vi "ArbitraryPlane_miniscan_Generator.vi"(8 "error in":errorcluster, 9 "Main Zoom":dbl, 10 "Frame Size":i32=200, 11 "Input data":T1(array[cluster])=[{"X start"=25.0, "Y start"=55.0, "Z start"=8.0}, {"X start"=96.0, "Y start"=109.0, "Z start"=5.0}, {"X start"=185.0, "Y start"=99.0, "Z start"=-10.0}]) -> (0 "error out":errorcluster, 1 "XYZ Stop Norm":cluster{"X":sgl, "Y":sgl, "Z":sgl}[](array[cluster]), 2 "XYZ Start Norm":cluster{"X":sgl, "Y":sgl, "Z":sgl}[](array[cluster]), 3 "Corners of Plane":dbl[][](array[numeric]), 4 "Number of pixels in single X miniscan":i32)   [LabVIEW 2020]
uses:
  Global Variables/gl_UI Ctrl Refs.vi
panel:
  out "XYZ Stop":cluster{"X":sgl, "Y":sgl, "Z":sgl}[](array[cluster])
  out "XYZ Start":cluster{"X":sgl, "Y":sgl, "Z":sgl}[](array[cluster])
  out "pixels in  tilted miniscan":sgl[](array[numeric])
  out "Debugging indicator":cluster{sgl, sgl}[](array[cluster])
  out "Number of miniscans":i32
  out "Ystop-Ystart":i32[](array[numeric])
  out "stops":sgl[][](array[numeric])
  out "starts":sgl[][](array[numeric])
  out "Number of pixels in each X miniscan":i32[](array[numeric])
  out "Path":path
  out "P3 (xyz)":dbl[](array[numeric])
  out "P2 (xyz)":dbl[](array[numeric])
  out "P1 (xyz)":dbl[](array[numeric])
  # "Columns are POI\n4 POI one for each rectangle corner."
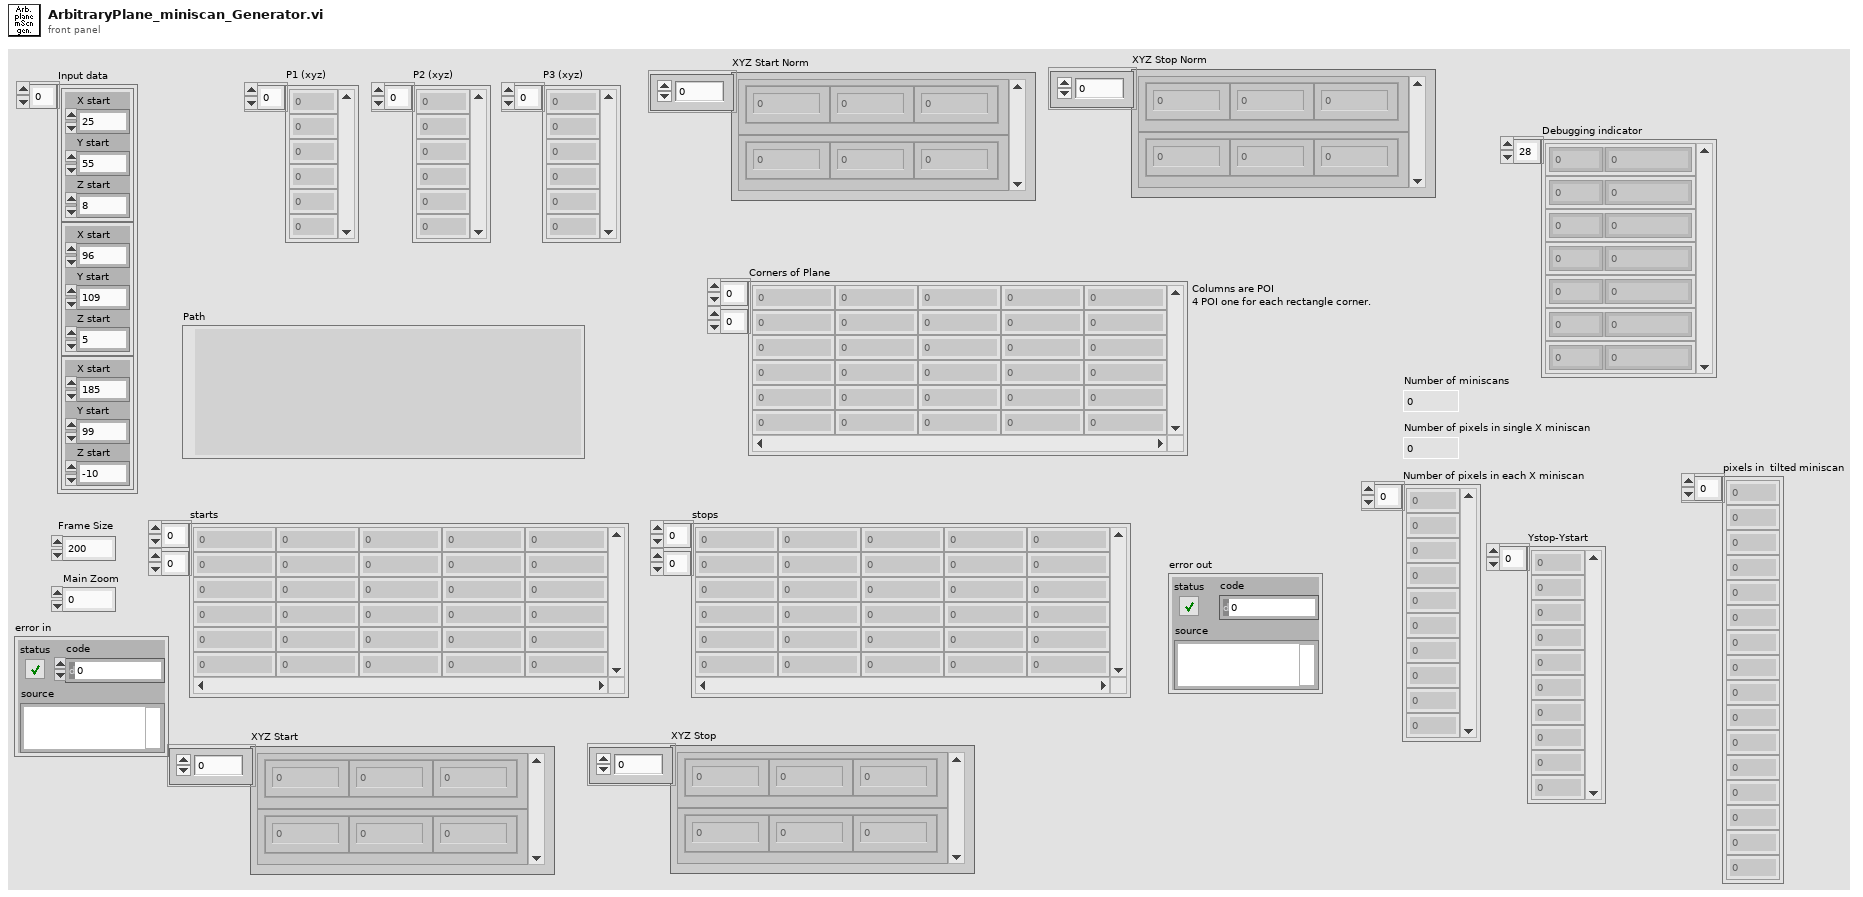
[diagram p1: front panel]
types:
  T1 = cluster{"X start":dbl, "Y start":dbl, "Z start":dbl}[]
  T2 = cluster{"X start":dbl, "Y start":dbl, "Z start":dbl}
  T3 = typedef "UI ctrl refs cluster.ctl" = cluster{"Top level VI path":path, "Top level VI ref":refnum<vi>, "User menu ref":refnum<k9>, "Sub Panel control":refnum<vi>, "Imaging Param Tab":refnum<vi>, "Occurrence-Start drivers":refnum<k4>, "Occurrence-Speed logging initialised":refnum<k4>, "Occurrence-XYZ stage initialised":refnum<k4>, "Exit button":refnum<vi>, "Status ind":refnum<vi>, "Set as origin":refnum<vi>, "Speed Logging":refnum<vi>, "Time Lapse":refnum<vi>, "Live Imaging":refnum<vi>, "AOL Z Stack":refnum<vi>, "Motor Z Stack":refnum<vi>, "Funct Acq button":refnum<vi>, "Hard Shutter":refnum<vi>, "Virtual Shutter":refnum<vi>, "Laser Power":refnum<vi>, "AOL Mode":refnum<vi>, "Frame Size":refnum<vi>, "Field of View":refnum<vi>, "Dwell Time":refnum<vi>, "Zoom":refnum<vi>, "AOL Z":refnum<vi>, "Objective":refnum<vi>, "Axis":refnum<vi>, "Paths & Names":refnum<vi>, "Experiment folder path (ind.)":refnum<vi>, "Last State (Ind.)":refnum<vi>, "Averages":refnum<vi>, "Angle (degrees)":refnum<vi>, "X centre":refnum<vi>, "Y centre":refnum<vi>, "Plane Mode":refnum<vi>, "# Planes":refnum<vi>, "Z Start":refnum<vi>, "Z Stop":refnum<vi>, "Z Step":refnum<vi>, "PMT 1":refnum<vi>, "PMT 2":refnum<vi>, "Stage XYZ Position":refnum<vi>, "Pockels@Z Start":refnum<vi>, "Pockels@Z Stop":refnum<vi>, "Obtain Z Start":refnum<vi>, "Obtain Z Stop":refnum<vi>, "Live stim.trig.period":refnum<vi>, "Live stim.trig.enable":refnum<vi>, "Movement Correction":refnum<vi>, "Load Reference Image":refnum<vi>, "XY Stage Move":refnum<vi>, "MovCor Cluster":refnum<vi>, "RefDAQParam":refnum<vi>, "Funct. Acq. Pockels Modulation":refnum<vi>, "Ref Laser Power":refnum<vi>, "Enable Video Recording":refnum<vi>, "Video Record-Live Imaging":refnum<vi>, "Video Record-Funct acq":refnum<vi>, "Reference Source":refnum<vi>, "AOL Z-stack Chirps Ready (ind)":refnum<vi>, "Target time between mov.cor. ref triggers (ms)":refnum<vi>, "Funct. Acq. Ref frame save":refnum<vi>, "Tracking button":refnum<vi>, "Show ref plots window":refnum<vi>, "Center freq ind (nm)":refnum<vi>, "Pickup mode (ind)":refnum<vi>, "Logging queue (ind)":refnum<vi>, "Back aperture power (ind.)":refnum<vi>, "Power after objective (ind.)":refnum<vi>, "Switch user":refnum<vi>, "Ls1 Conn. Status":refnum<vi>, "Ls1Tuning Status":refnum<vi>, "Ls1 Faults":refnum<vi>, "Ls1 Connection":refnum<vi>, "Ls1 Mode":refnum<vi>, "Ls1 POWER [mW]":refnum<vi>, "Ls1Shutter":refnum<vi>, "Ls1 Wavelength":refnum<vi>, "Ls1 Note":refnum<vi>, "Ls1 Confirm Wav":refnum<vi>, "Ls1 PreChrp Prism1":refnum<vi>, "Ls1 PreChrp Prism2":refnum<vi>, "Ls1 wav top Ind":refnum<vi>, "Ls1 power top Ind":refnum<vi>, "Ls1 Pump peak Hold":refnum<vi>, "Ls1 Status Ind":refnum<vi>, "Ls1 wav cancel":refnum<vi>, "Experiment Type":refnum<vi>, "Biology Information":refnum<vi>, "Camera recording status":refnum<vi>}
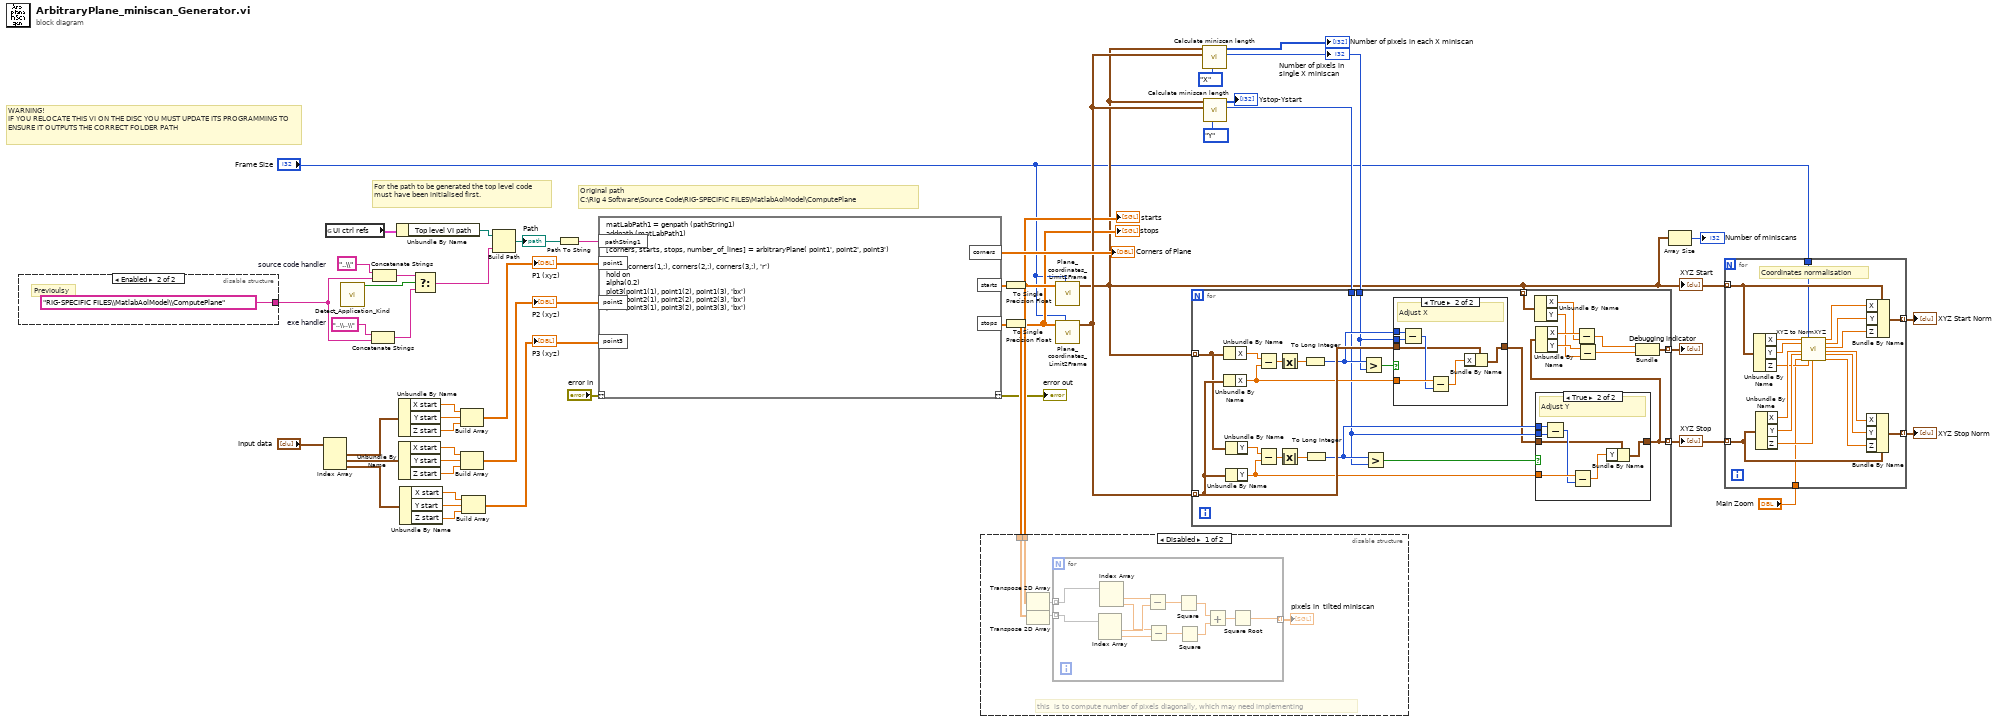
[diagram p0: block diagram]
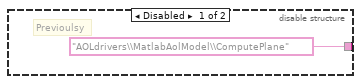
[diagram p2: hidden frame]
diagram:
  w6 = "..\\"  # source code handler
  w7 = "..\\..\\"  # exe handler
  # "WARNING!\nIF YOU RELOCATE THIS VI ON THE DISC YOU MUST UPDATE ITS PROGRAMMING TO ENSURE IT OUTPUTS THE CORRECT FOLDER PATH"
  # "For the path to be generated the top level code must have been initialised first."
  # "Original path\nC:\\Rig 4 Software\\Source Code\\RIG-SPECIFIC FILES\\MatlabAolModel\\ComputePlane"
  n1 = disable-structure shown="Enabled" {
    disable-tunnel: ["AOLdrivers\\MatlabAolModel\\ComputePlane" "RIG-SPECIFIC FILES\\MatlabAolModel\\ComputePlane"] -> w5
    frame Disabled {
      # "Previoulsy"
    }
    frame Enabled {
      # "Previoulsy"
    }
  }
  n2 = Index Array(array="Input data") -> (element #1=w41:T2, element #2=w30:T2, element #3=w29:T2)  [unwired: 3 in]
  n3 = global read "gl_UI Ctrl Refs.vi" "UI ctrl refs"() -> (w44:T3)
  n4 = call <userlib>:"Detect_Application_Kind.vi"() -> ("Development System"=w9:bool)  [unwired: 9 in, 2 out]
  n5 = Concatenate Strings(w7, w5) -> (w8:string)
  n6 = Concatenate Strings(w6, w5) -> (w4:string)
  n7 = Unbundle By Name(w44) -> ("Top level VI path"=w45:path)
  n8 = Unbundle By Name(w41) -> ("X start"=w40:dbl, "Y start"=w38:dbl, "Z start"=w39:dbl)
  n9 = Unbundle By Name(w30) -> ("X start"=w34:dbl, "Y start"=w36:dbl, "Z start"=w35:dbl)
  n10 = Unbundle By Name(w29) -> ("X start"=w33:dbl, "Y start"=w31:dbl, "Z start"=w32:dbl)
  n11 = Select(t=w4, s=w9, f=w8) -> (s? t:f=w10:string)
  n12 = Build Array(w40, w38, w39) -> (w37:dbl[])
  "P1 (xyz)" <- w37
  n13 = Build Array(w34, w36, w35) -> (w27:dbl[])
  "P2 (xyz)" <- w27
  n14 = Build Array(w33, w31, w32) -> (w28:dbl[])
  "P3 (xyz)" <- w28
  n15 = Build Path(base path=w45, name or relative path=w10) -> (appended path=w43:path)
  "Path" <- w43
  n16 = Path To String(path=w43) -> (string=w42:string)
  n17 = script code="matLabPath1 = genpath (pathString1)\naddpath (matLabPath1)\n\n[corners, starts, stops, number_of_lines] = arbitraryPlane( point1', point2', point3')\n\npatch(corners(1,:), corners(2,:), corners(3,:), 'r')\nhold on\nalpha(0.2)\nplot3(point1(1), point1(2), point1(3), 'bx')\nplot3(point2(1), point2(2), point2(3), 'bx')\nplot3(point3(1), point3(2), point3(3), 'bx')" ("Script Node")("??"="error in", "point1"=w37, "point2"=w27, "point3"=w28, "pathString1"=w42) -> ("??"=→"error out":errorcluster, "corners"=→"Corners of Plane":dbl[][], "starts"=w48:dbl[][], "stops"=w47:dbl[][])
  n18 = To Single Precision Float(number=w48) -> (single precision float=w17:sgl[][])
  "starts" <- w17
  n19 = To Single Precision Float(number=w47) -> (single precision float=w16:sgl[][])
  "stops" <- w16
  n20 = disable-structure shown="Disabled" {
    disable-tunnel: w17 -> [w56 _]
    disable-tunnel: w16 -> [w55 _]
    frame Disabled {
      # "this  is to compute number of pixels diagonally, which may need implementing"
      n21 = Transpose 2D Array(2D array=w56) -> (transposed array=w54:sgl[][])
      n22 = Transpose 2D Array(2D array=w55) -> (transposed array=w53:sgl[][])
      n23 = for {
        tunnel: w54 -> [w68] mode=indexing
        tunnel: w53 -> [w67] mode=indexing
        tunnel: [w57] -> w52 mode=indexing
        n24 = Index Array(array=w67) -> (element #1=w65:sgl, element #2=w63:sgl)  [unwired: 2 in]
        n25 = Index Array(array=w68) -> (element #1=w66:sgl, element #2=w64:sgl)  [unwired: 2 in]
        n26 = Subtract(x=w66, y=w65) -> (x-y=w62:sgl)
        n27 = Subtract(x=w64, y=w63) -> (x-y=w61:sgl)
        n28 = Square(x=w62) -> (x^2=w59:sgl)
        n29 = Square(x=w61) -> (x^2=w60:sgl)
        n30 = Add(x=w59, y=w60) -> (x+y=w58:sgl)
        n31 = Square Root(x=w58) -> (sqrt(x)=w57:sgl)
      }
      "pixels in  tilted miniscan" <- w52
    }
    frame Enabled {
    }
  }
  n32 = call "Plane_coordinates_Limit2Frame.vi"("Frame Size"="Frame Size", "Input Array"=w17) -> ("XYZ Start"=w15:cluster{"X":sgl, "Y":sgl, "Z":sgl}[])  [unwired: 9 in]
  "XYZ Start" <- w15
  n33 = call "Plane_coordinates_Limit2Frame.vi"("Frame Size"="Frame Size", "Input Array"=w16) -> ("XYZ Start"=w23:cluster{"X":sgl, "Y":sgl, "Z":sgl}[])  [unwired: 9 in]
  n34 = call "Calculate miniscan length.vi"("Enum"=enum16{"X", "Y"}."X", "XYZ Stop"=w23, "XYZ Start"=w15) -> ("Number of pixels in single miniscan"=w20:i32, "Number of pixels in each miniscan"=→"Number of pixels in each X miniscan":i32[])  [unwired: 7 in]
  "Number of pixels in single X miniscan" <- w20
  n35 = call "Calculate miniscan length.vi"("Enum"=enum16{"X", "Y"}."Y", "XYZ Stop"=w23, "XYZ Start"=w15) -> ("Number of pixels in single miniscan"=w19:i32, "Number of pixels in each miniscan"=→"Ystop-Ystart":i32[])  [unwired: 7 in]
  n36 = for {
    tunnel: w15 -> [w78] mode=indexing
    tunnel: w23 -> [w87] mode=indexing
    tunnel: w20 -> [w85]
    tunnel: w19 -> [w80]
    tunnel: [w69] -> w14 mode=indexing
    tunnel: [w71] -> w24 mode=indexing
    tunnel: w15 -> [w70] mode=indexing
    n37 = Unbundle By Name(w78) -> ("X"=w93:sgl)
    n38 = Unbundle By Name(w87) -> ("X"=w84:sgl)
    n39 = Unbundle By Name(w78) -> ("Y"=w91:sgl)
    n40 = Unbundle By Name(w87) -> ("Y"=w82:sgl)
    n41 = Subtract(x=w93, y=w84) -> (x-y=w94:sgl)
    n42 = Subtract(x=w91, y=w82) -> (x-y=w92:sgl)
    n43 = Absolute Value(x=w94) -> (abs(x)=w90:sgl)
    n44 = Absolute Value(x=w92) -> (abs(x)=w89:sgl)
    n45 = To Long Integer(number=w90) -> (32bit integer=w86:i32)
    n46 = To Long Integer(number=w89) -> (32bit integer=w81:i32)
    n47 = Greater?(x=w86, y=w85) -> (0:w88:bool)
    n48 = Greater?(x=w81, y=w80) -> (0:w83:bool)
    n49 = case shown="True" w88 {
      tunnel: w87 -> [w103 w106]
      tunnel: [w103 w104] -> w79
      tunnel: w86 -> [_ w110]
      tunnel: w85 -> [_ w109]
      tunnel: w84 -> [_ w108]
      frame False {
      }
      frame True {
        # "Adjust X"
        n50 = Subtract(x=w110, y=w109) -> (x-y=w107:i32)
        n51 = Subtract(x=w108, y=w107) -> (x-y=w105:sgl)
        n52 = Bundle By Name(cluster=w106, "X"=w105) -> (w104:cluster{"X":sgl, "Y":sgl, "Z":sgl})
      }
    }
    n53 = Unbundle By Name(w70) -> ("X"=w76:sgl, "Y"=w74:sgl)
    n54 = case shown="True" w83 {
      tunnel: w79 -> [w95 w98]
      tunnel: [w95 w96] -> w69
      tunnel: w81 -> [_ w102]
      tunnel: w80 -> [_ w101]
      tunnel: w82 -> [_ w100]
      frame False {
      }
      frame True {
        # "Adjust Y"
        n55 = Subtract(x=w102, y=w101) -> (x-y=w99:i32)
        n56 = Subtract(x=w100, y=w99) -> (x-y=w97:sgl)
        n57 = Bundle By Name(cluster=w98, "Y"=w97) -> (w96:cluster{"X":sgl, "Y":sgl, "Z":sgl})
      }
    }
    n58 = Unbundle By Name(w69) -> ("X"=w77:sgl, "Y"=w75:sgl)
    n59 = Subtract(x=w77, y=w76) -> (x-y=w73:sgl)
    n60 = Subtract(x=w75, y=w74) -> (x-y=w72:sgl)
    n61 = Bundle(w73, w72) -> (w71:cluster{sgl, sgl})  [unwired: 1 in]
  }
  "Debugging indicator" <- w24
  "XYZ Stop" <- w14
  n62 = Array Size(array=w15) -> (size(s)=→"Number of miniscans":i32)
  n63 = for {
    tunnel: w15 -> [w122] mode=indexing
    tunnel: w14 -> [w117] mode=indexing
    tunnel: [w121] -> w13 mode=indexing
    tunnel: [w113] -> w12 mode=indexing
    tunnel: "Frame Size" -> [w112]
    tunnel: "Main Zoom" -> [w111]
    # "Coordinates normalisation"
    n64 = Unbundle By Name(w122) -> ("X"=w128:sgl, "Y"=w127:sgl, "Z"=w124:sgl)
    n65 = Unbundle By Name(w117) -> ("X"=w126:sgl, "Y"=w125:sgl, "Z"=w123:sgl)
    n66 = call "XYZ to NormXYZ.vi"("X start"=w128, "Y start"=w127, "X stop"=w126, "Y stop"=w125, "Zoom (either ref or main zoom)"=w111, "FrameSize"=w112, "Z start"=w124, "Z stop"=w123) -> ("Norm X Start"=w120:dbl, "Norm Y Start"=w119:dbl, "Norm Z Start"=w118:dbl, "Norm X Stop"=w116:dbl, "Norm Y Stop"=w115:dbl, "Norm Z Stop"=w114:dbl)  [unwired: 6 in]
    n67 = Bundle By Name(cluster=w117, "X"=w116, "Y"=w115, "Z"=w114) -> (w113:cluster{"X":sgl, "Y":sgl, "Z":sgl})
    n68 = Bundle By Name(cluster=w122, "X"=w120, "Y"=w119, "Z"=w118) -> (w121:cluster{"X":sgl, "Y":sgl, "Z":sgl})
  }
  "XYZ Start Norm" <- w13
  "XYZ Stop Norm" <- w12
